vi "Raster Scan.vi"() -> ()   [LabVIEW 2012]
uses:
  Madlib.dll
panel:
  in  "XRasterRead":dbl[](array[numeric])
  in  "YRasterRead":dbl[](array[numeric])
  in  "ZRasterRead":dbl[](array[numeric])
  in  "Tab Control":T1(tab)
  in  "exportData":bool
  out "Actual Total Time":dbl format="%#.3f"
  in  "commandZ":bool
  in  "commandY":bool
  out "zRead":dbl format="%#.3g"
  out "yRead":dbl format="%#.3g"
  out "xRead":dbl format="%#.3g"
  in  "zCommand":dbl
  in  "yCommand":dbl
  in  "xCommand":dbl
  out "XY Graph":cluster{"Y":dbl[], "Y":dbl[]}[](graph)
  in  "pixel read delay":dbl=5.0
  in  "pixels reads per line":dbl=10.0
  in  "startScan":bool
  in  "3D Raster Scan":bool
  in  "mirroredMotion":bool
  in  "waveAcquistion":bool
  in  "frame delay":dbl=50.0
  in  "end of line delay":dbl=50.0
  in  "start of line delay":dbl=50.0
  in  "pixel write delay":dbl=5.0
  in  "Zend":dbl=1.0
  in  "Zstart":dbl
  in  "frames per scan":dbl=5.0
  in  "Yend":dbl=1.0
  in  "Ystart":dbl
  in  "lines per frame":dbl=10.0
  in  "pixels writes per line":dbl=20.0
  in  "Xend":dbl=1.0
  in  "Xstart":dbl
  in  "init handle":bool
  out "handle found":bool
  in  "Y-Axis Display":u8(ring)=2 items=["Point by Point", "Line", "Pixel"]
  in  "X-Axis Display":u8(ring) items=["Point by Point", "Line", "Pixel"]
  in  "stop":bool
  in  "commandX":bool
  out "Expected Total Time":dbl format="%#_6f"
  in  "exportDataSelect":u8(ring)=2 items=["ADC (blue) as graphed", "DAC (green) as graphed", "First and last ADC dpt of each line", "All pixel ADC", "All line ADC", "All frame ADC", "All pixel DAC", "All line DAC", "All frame DAC"]
  in  "Frame":u32=1 min=1
  in  "View Start of Scan ISS Commands":bool caption="View End of Scan ISS Commands"
  in  "Adv ISS Control":bool
  in  "ISSConfirm":bool
  in  "ISSReset":bool
  in  "AuxBindAxis":T2(ring)
  in  "AuxPulse":enum16{"Low to High", "High to Low"}(ring)
  in  "AuxPol":enum16{"Low", "High"}(ring)
  in  "FrameBindAxis":T2(ring)
  in  "FramePulse":enum16{"Low to High", "High to Low"}(ring)
  in  "FramePol":enum16{"Low", "High"}(ring)
  in  "LineBindAxis":T2(ring)
  in  "LinePulse":enum16{"Low to High", "High to Low"}(ring)
  in  "LinePol":enum16{"Low", "High"}(ring)
  in  "PixRestore":bool
  in  "PixBindAxis":T2(ring)
  in  "PixPulse":enum16{"Low to High", "High to Low"}(ring)
  in  "PixPol":enum16{"Low", "High"}(ring)
  in  "LineRestore":bool
  in  "FrameRestore":bool
  in  "AuxRestore":bool
  in  "PulseAux":bool
  in  "PulseFrame":bool
  in  "PulseLine":bool
  in  "PulsePix":bool
  out "zPos":dbl[](graph)
  out "yPos":dbl[](graph)
  out "xPos":dbl[](graph)
  # "Step 1: Initialize an MCL device"
  # "Step 6: Define the Scan Timing"
  # "ms"
  # "ms"
  # "ms"
  # "Step 2: Use the \"ISS Config.\" tab to set\n             up and test the ISS option."
  # "ms"
  # "ms"
  # "Step 3: Choose how to perform the scan"
  # "Step 7: Run the scan"
  # "use waveform acquisition \n(16-bit NanoDrive)"
  # "pixel axis mirrors\nmotion on return"
  # "3-D raster scan"
  # "s"
  # "Step 4: Define the region to scan"
  # "s"
  # "Nano-Drive X-Axis (pixel) scan region"
  # "Step 8: Export the data"
  # "start"
  # "um"
  # "end"
  # "um"
  # "Nano-Drive Y-Axis (line) scan region"
  # "generates a file with 2 columns of data; the left containing the graph's; X-axis, the right containing the graph'sY-axis."
  # "*"
  # "start"
  # "um"
  # "end"
  # "um"
  # "Nano-Drive Z-Axis (frame) scan region"
  # "Step 9: Release the MCL device and\n              end the VI."
  # "start"
  # "um"
  # "end"
  # "um"
  # "Step 5: Define the Scan Resolution"
  # "Graph Configuration"
  # "Current Positions"
  # "X axis"
  # "Y axis"
  # "Z axis"
  # "ISS Configuration"
  # "Pixel Clock"
  # "Line Clock"
  # "Frame Clock"
  # "Auxilary Clock"
  # "* Only one clock can be bound to an axis or event. Binding a second clock\n    replaces the first with the second"
  # "Confirm/Reset \nISS Configuration:"
  # "* Changes made here take no effect until confirmed."
  # "* Binding a Clock to an Axis will result in the suspension of live\n  position reads."
  # "Programmatic ISS Control"
  # "Pulse Individual \nISS Clocks:"
  # "* Pulsing will reset Clock to Low polarity."
  # "X\n\na\nx\ni\ns"
  # "Y\n\na\nx\ni\ns"
  # "Z\n\na\nx\ni\ns"
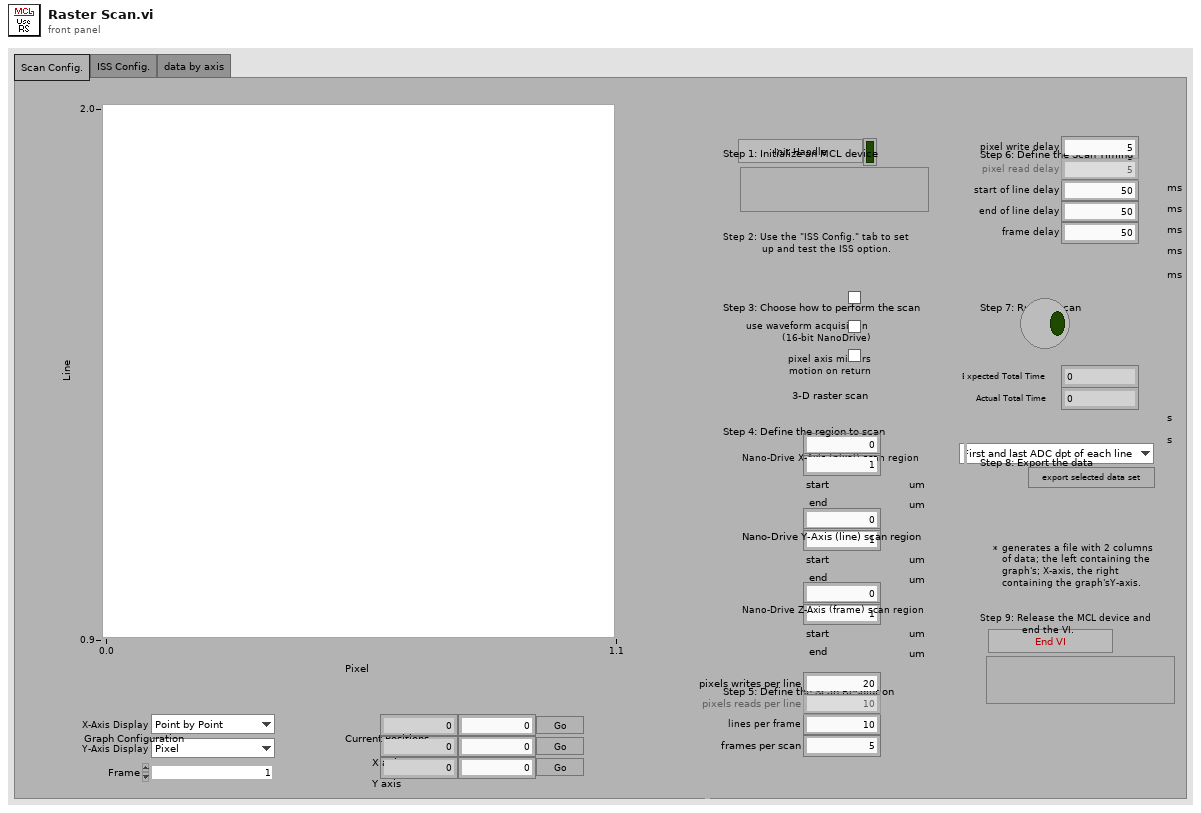
[diagram p1: front panel]
types:
  T1 = enum32{"Scan Config.", "ISS Config.", "data by axis"}
  T2 = enum16{"Unbound", "X Axis", "Y Axis", "Z Axis", "Auxilary", "Waveform Read", "Waveform Write"}
  T3 = cluster{"ISSReset":bool, "Pixel Confirmed Options":cluster{"clock (1=Pixel)":i32, "Pixel Polarity":enum16{"Low", "High"}, "Pixel Pulse":enum16{"Low to High", "High to Low"}, "Pixel Bind":enum16{"Unbound", "X Axis", "Y Axis", "Z Axis", "Auxilary", "Waveform Read", "Waveform Write"}}, "Line Confirmed Options":cluster{"clock (1=Pixel)":i32, "Pixel Polarity":enum16{"Low", "High"}, "Pixel Pulse":enum16{"Low to High", "High to Low"}, "Pixel Bind":enum16{"Unbound", "X Axis", "Y Axis", "Z Axis", "Auxilary", "Waveform Read", "Waveform Write"}}, "Frame Confirmed Options":cluster{"clock (1=Pixel)":i32, "Pixel Polarity":enum16{"Low", "High"}, "Pixel Pulse":enum16{"Low to High", "High to Low"}, "Pixel Bind":enum16{"Unbound", "X Axis", "Y Axis", "Z Axis", "Auxilary", "Waveform Read", "Waveform Write"}}, "Aux Confirmed Options":cluster{"clock (1=Pixel)":i32, "Pixel Polarity":enum16{"Low", "High"}, "Pixel Pulse":enum16{"Low to High", "High to Low"}, "Pixel Bind":enum16{"Unbound", "X Axis", "Y Axis", "Z Axis", "Auxilary", "Waveform Read", "Waveform Write"}}}
  T4 = cluster{"waveAcquistion":bool, "mirroredMotion":bool, "3D Raster Scan":bool}
  T5 = cluster{"Xstart":dbl, "Xend":dbl, "Ystart":dbl, "Yend":dbl, "Zstart":dbl, "Zend":dbl}
  T6 = cluster{"pixels writes per line":dbl, "pixels reads per line":dbl, "lines per frame":dbl, "frames per scan":dbl}
  T7 = cluster{"pixel write delay":dbl, "pixel read delay":dbl, "start of line delay":dbl, "end of line delay":dbl, "frame delay":dbl}
  T8 = cluster{"exportDataSelect":u8, "exportData":bool}
  T9 = cluster{"X-Axis Display":u8, "Y-Axis Display":u8, u32}
  T10 = cluster{cluster{"waveAcquistion":bool, "mirroredMotion":bool, "3D Raster Scan":bool}, cluster{"Xstart":dbl, "Xend":dbl, "Ystart":dbl, "Yend":dbl, "Zstart":dbl, "Zend":dbl}, cluster{"pixels writes per line":dbl, "pixels reads per line":dbl, "lines per frame":dbl, "frames per scan":dbl}, cluster{"pixel write delay":dbl, "pixel read delay":dbl, "start of line delay":dbl, "end of line delay":dbl, "frame delay":dbl}}
  T11 = cluster{"XY Graph":refnum<vi>, cluster{"exportDataSelect":u8, "exportData":bool}, cluster{"X-Axis Display":u8, "Y-Axis Display":u8, u32}}
  T12 = cluster{"PixRestore":bool, "LineRestore":bool, "FrameRestore":bool, "AuxRestore":bool}
  T13 = cluster{"PixBindAxis":enum16{"Unbound", "X Axis", "Y Axis", "Z Axis", "Auxilary", "Waveform Read", "Waveform Write"}, "LineBindAxis":enum16{"Unbound", "X Axis", "Y Axis", "Z Axis", "Auxilary", "Waveform Read", "Waveform Write"}, "FrameBindAxis":enum16{"Unbound", "X Axis", "Y Axis", "Z Axis", "Auxilary", "Waveform Read", "Waveform Write"}, "AuxBindAxis":enum16{"Unbound", "X Axis", "Y Axis", "Z Axis", "Auxilary", "Waveform Read", "Waveform Write"}}
  T14 = cluster{"PixPol":enum16{"Low", "High"}, "PixPulse":enum16{"Low to High", "High to Low"}, "LinePol":enum16{"Low", "High"}, "LinePulse":enum16{"Low to High", "High to Low"}, "FramePol":enum16{"Low", "High"}, "FramePulse":enum16{"Low to High", "High to Low"}, "AuxPol":enum16{"Low", "High"}, "AuxPulse":enum16{"Low to High", "High to Low"}}
  T15 = cluster{"PulsePix":bool, "PulseLine":bool, "PulseFrame":bool, "PulseAux":bool}
  T16 = cluster{"ISS Options":cluster{"ISSReset":bool, "Pixel Confirmed Options":cluster{"clock (1=Pixel)":i32, "Pixel Polarity":enum16{"Low", "High"}, "Pixel Pulse":enum16{"Low to High", "High to Low"}, "Pixel Bind":enum16{"Unbound", "X Axis", "Y Axis", "Z Axis", "Auxilary", "Waveform Read", "Waveform Write"}}, "Line Confirmed Options":cluster{"clock (1=Pixel)":i32, "Pixel Polarity":enum16{"Low", "High"}, "Pixel Pulse":enum16{"Low to High", "High to Low"}, "Pixel Bind":enum16{"Unbound", "X Axis", "Y Axis", "Z Axis", "Auxilary", "Waveform Read", "Waveform Write"}}, "Frame Confirmed Options":cluster{"clock (1=Pixel)":i32, "Pixel Polarity":enum16{"Low", "High"}, "Pixel Pulse":enum16{"Low to High", "High to Low"}, "Pixel Bind":enum16{"Unbound", "X Axis", "Y Axis", "Z Axis", "Auxilary", "Waveform Read", "Waveform Write"}}, "Aux Confirmed Options":cluster{"clock (1=Pixel)":i32, "Pixel Polarity":enum16{"Low", "High"}, "Pixel Pulse":enum16{"Low to High", "High to Low"}, "Pixel Bind":enum16{"Unbound", "X Axis", "Y Axis", "Z Axis", "Auxilary", "Waveform Read", "Waveform Write"}}}, cluster{"ISSConfirm":bool, "ISSReset":bool}, cluster{"PixRestore":bool, "LineRestore":bool, "FrameRestore":bool, "AuxRestore":bool}, cluster{"PixBindAxis":enum16{"Unbound", "X Axis", "Y Axis", "Z Axis", "Auxilary", "Waveform Read", "Waveform Write"}, "LineBindAxis":enum16{"Unbound", "X Axis", "Y Axis", "Z Axis", "Auxilary", "Waveform Read", "Waveform Write"}, "FrameBindAxis":enum16{"Unbound", "X Axis", "Y Axis", "Z Axis", "Auxilary", "Waveform Read", "Waveform Write"}, "AuxBindAxis":enum16{"Unbound", "X Axis", "Y Axis", "Z Axis", "Auxilary", "Waveform Read", "Waveform Write"}}, cluster{"PixPol":enum16{"Low", "High"}, "PixPulse":enum16{"Low to High", "High to Low"}, "LinePol":enum16{"Low", "High"}, "LinePulse":enum16{"Low to High", "High to Low"}, "FramePol":enum16{"Low", "High"}, "FramePulse":enum16{"Low to High", "High to Low"}, "AuxPol":enum16{"Low", "High"}, "AuxPulse":enum16{"Low to High", "High to Low"}}, cluster{"PulsePix":bool, "PulseLine":bool, "PulseFrame":bool, "PulseAux":bool}, "handle":i32}
  T17 = cluster{"XRasterRead":dbl[], "YRasterRead":dbl[], "ZRasterRead":dbl[]}
  T18 = cluster{"stop":refnum<vi>, "startScan":refnum<vi>, "Adv ISS Control":bool}
  T19 = cluster{refnum<vi>, "handle":i32, "OwningVI":refnum<vi>}
  T20 = cluster{"reset pixel":bool, "reset line":bool, "reset frame":bool, "reset aux":bool}
  T21 = cluster{cluster{"stop":refnum<vi>, "startScan":refnum<vi>, "Adv ISS Control":bool}, cluster{refnum<vi>, "handle":i32, "OwningVI":refnum<vi>}}
  T22 = cluster{"X Command Ramp":dbl[], "Y Command Ramp":dbl[], "Z Command Ramp":dbl[]}
  T23 = cluster{"Options":cluster{"waveAcquistion":bool, "mirroredMotion":bool, "3DRasterScan":bool}, "Regions":cluster{"xStart":dbl, "xEnd":dbl, "yStart":dbl, "yEnd":dbl, "zStart":dbl, "zEnd":dbl}, "Resolution":cluster{"pixelsWritesPerLine":dbl, "pixelsReadsPerLine":dbl, "linesPerFrame":dbl, "framesPerScan":dbl}, "Timing":cluster{"pixelWriteDelay":dbl, "pixelReadDelay":dbl, "startOfLineDelay":dbl, "endOfLineDelay":dbl, "frameDelay":dbl}}
  T24 = cluster{refnum<vi>[], refnum<vi>[], refnum<vi>[]}
  T25 = cluster{"clock (1=Pixel)":i32, "Pixel Polarity":enum16{"Low", "High"}, "Pixel Pulse":enum16{"Low to High", "High to Low"}, "Pixel Bind":enum16{"Unbound", "X Axis", "Y Axis", "Z Axis", "Auxilary", "Waveform Read", "Waveform Write"}}
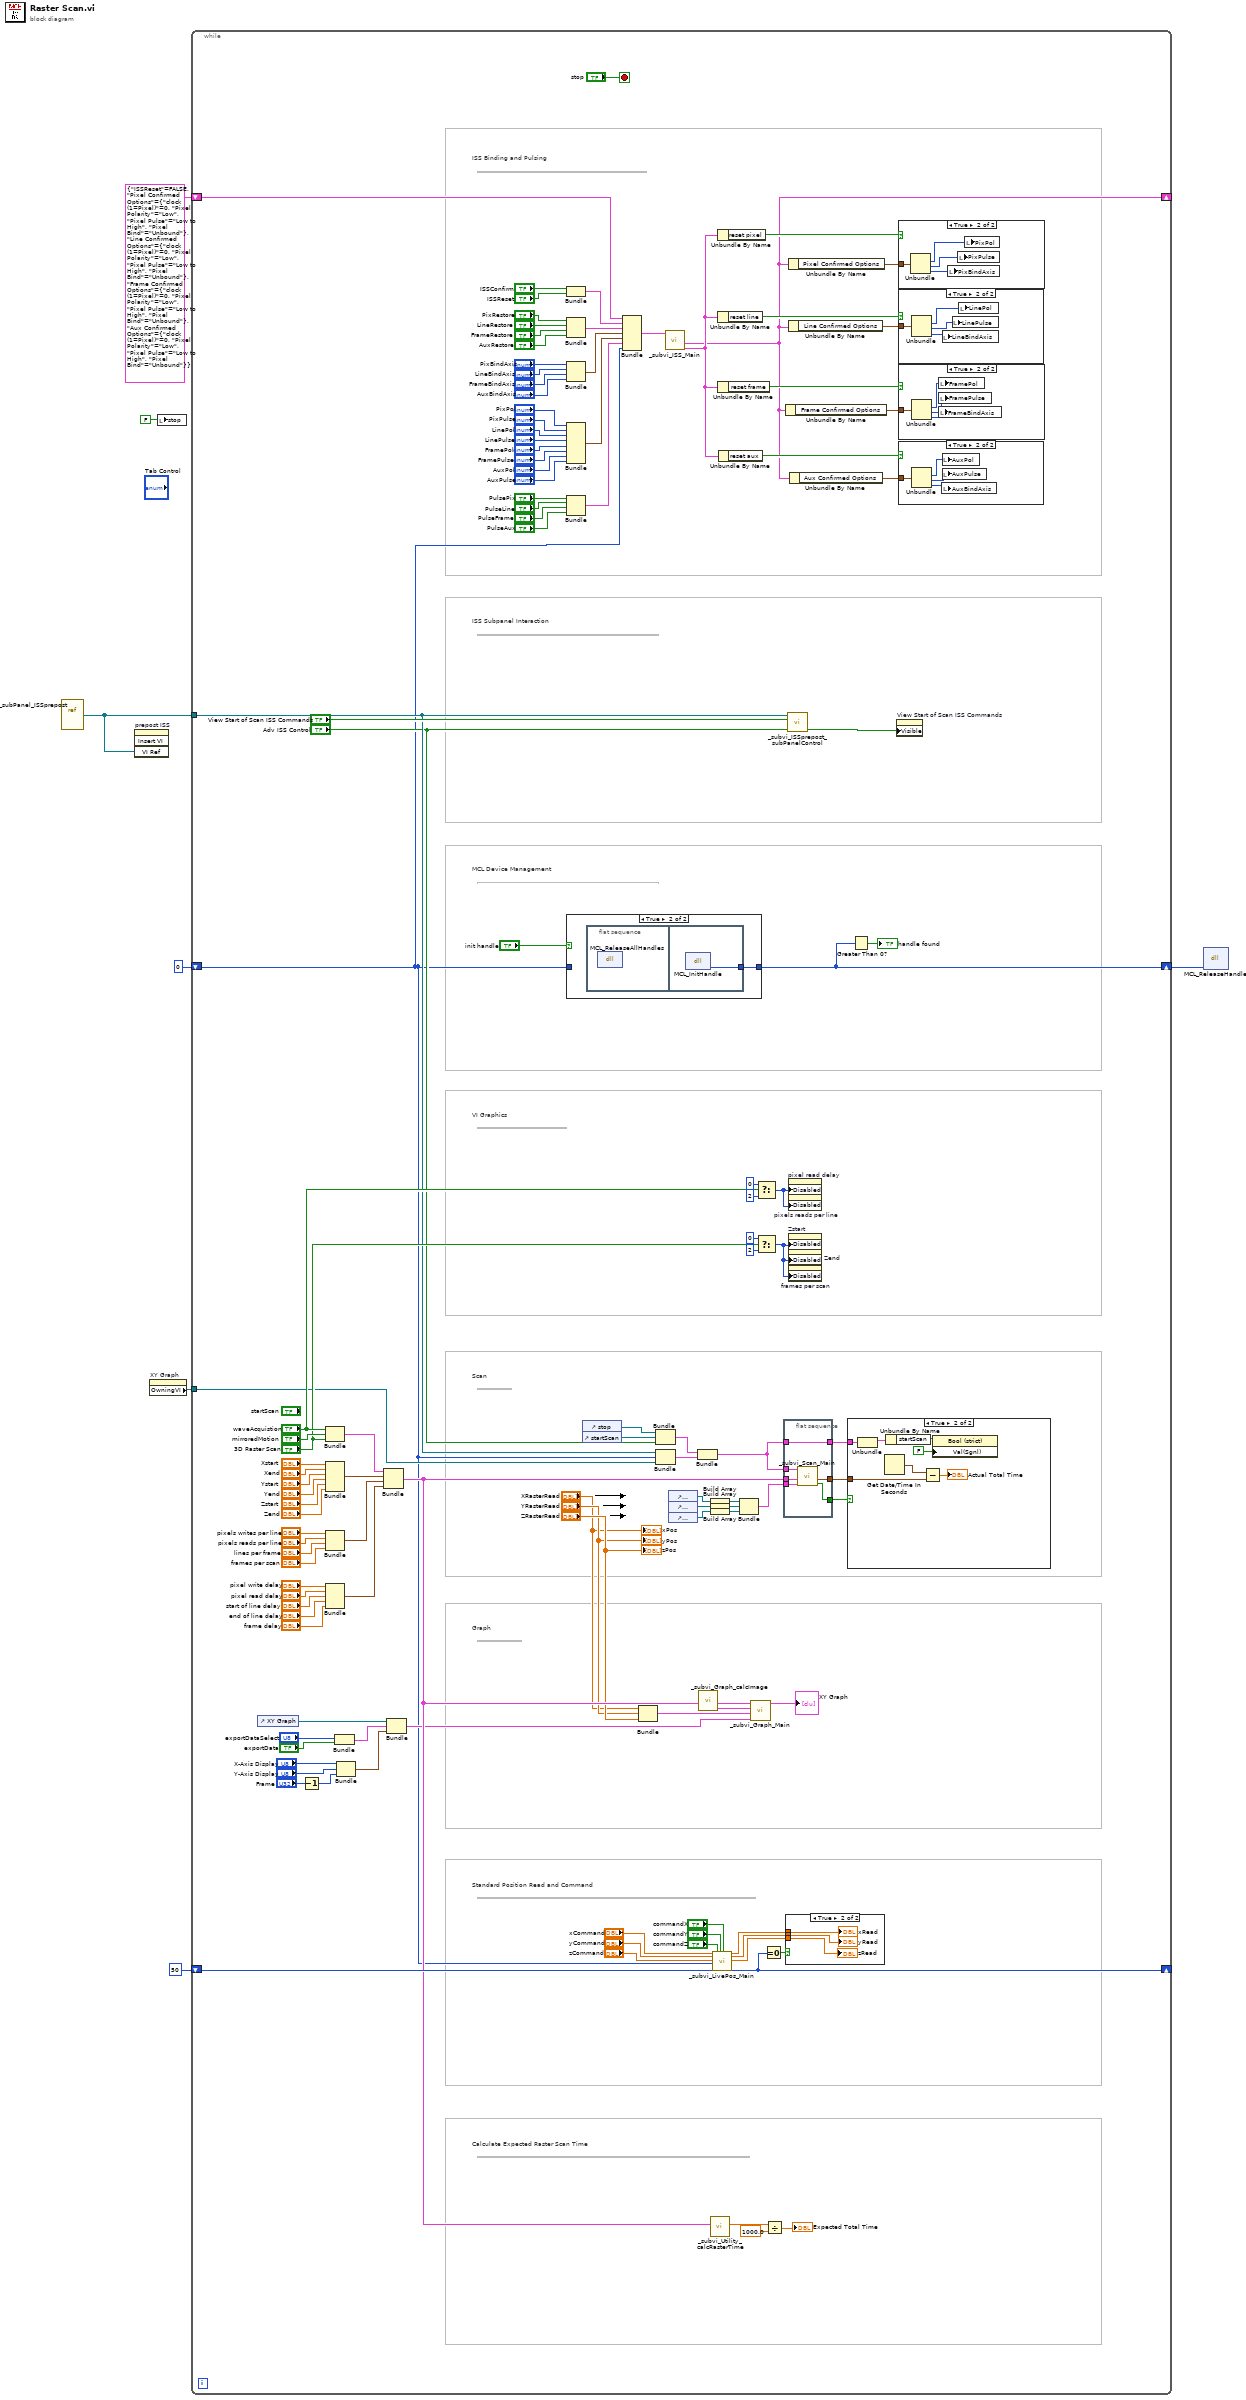
[diagram p0: block diagram]
diagram:
  n1 = vi-ref "_subPanel_ISSprepost.vi"() -> (w5:refnum<vi>)
  n2 = invoke on="prepost ISS" class="SubPanel" method="Insert VI"("VI Ref"=w5) -> ()  [unwired: 3 in, 4 out]
  n3 = property on="XY Graph" class="XYGraph (strict)"() -> ("OwningVI"=w2:refnum<vi>)  [unwired: 2 in, 2 out]
  n4 = local write "stop"(FALSE ("stop")) -> ()
  n5 = while {
    shift-right: [w95] -> _
    shift-left: T3 {"ISSReset"=FALSE, "Pixel Confirmed Options"={"clock (1=Pixel)"=0, "Pixel Polarity"=enum."Low", "Pixel Pulse"=enum."Low to High", "Pixel Bind"=enum."Unbound"}, "Line Confirmed Options"={"clock (1=Pixel)"=0, "Pixel Polarity"=enum."Low", "Pixel Pulse"=enum."Low to High", "Pixel Bind"=enum."Unbound"}, "Frame Confirmed Options"={"clock (1=Pixel)"=0, "Pixel Polarity"=enum."Low", "Pixel Pulse"=enum."Low to High", "Pixel Bind"=enum."Unbound"}, "Aux Confirmed Options"={"clock (1=Pixel)"=0, "Pixel Polarity"=enum."Low", "Pixel Pulse"=enum."Low to High", "Pixel Bind"=enum."Unbound"}} ("ISS Options") -> [w61]
    tunnel: w5 -> [w56]
    shift-right: [w89] -> w4
    shift-left: 0 ("handle") -> [w8]
    tunnel: w2 -> [w54]
    shift-right: [w31] -> _
    shift-left: u32 50 ("axis") -> [w33]
    stop <- "stop" stop-if-true
    # "Calculate Expected Raster Scan Time"
    # "Standard Position Read and Command"
    # "Graph"
    # "Scan"
    # "VI Graphics"
    # "MCL Device Management"
    # "ISS Subpanel Interaction"
    # "ISS Binding and Pulsing"
    n6 = control-ref of="XY Graph"() -> (w60:refnum<vi>)
    n7 = Decrement(x="Frame") -> (x-1=w10:u32)
    n8 = Bundle("waveAcquistion"="waveAcquistion", "mirroredMotion"="mirroredMotion", "3D Raster Scan"="3D Raster Scan") -> (w65:T4)  [unwired: 1 out]
    n9 = Bundle("Xstart"="Xstart", "Xend"="Xend", "Ystart"="Ystart", "Yend"="Yend", "Zstart"="Zstart", "Zend"="Zend") -> (w64:T5)  [unwired: 1 out]
    n10 = Bundle("pixels writes per line"="pixels writes per line", "pixels reads per line"="pixels reads per line", "lines per frame"="lines per frame", "frames per scan"="frames per scan") -> (w63:T6)  [unwired: 1 out]
    n11 = Bundle("pixel write delay"="pixel write delay", "pixel read delay"="pixel read delay", "start of line delay"="start of line delay", "end of line delay"="end of line delay", "frame delay"="frame delay") -> (w62:T7)  [unwired: 1 out]
    n12 = Bundle("exportDataSelect"="exportDataSelect", "exportData"="exportData") -> (w24:T8)  [unwired: 1 out]
    n13 = Bundle("X-Axis Display"="X-Axis Display", "Y-Axis Display"="Y-Axis Display", w10) -> (w27:T9)  [unwired: 1 out]
    n14 = Bundle(w65, w64, w63, w62) -> (w19:T10)  [unwired: 1 out]
    n15 = Bundle("XY Graph"=w60, w24, w27) -> (w16:T11)  [unwired: 1 out]
    n16 = Bundle("ISSConfirm"="ISSConfirm", "ISSReset"="ISSReset") -> (w101:cluster{"ISSConfirm":bool, "ISSReset":bool})  [unwired: 1 out]
    n17 = Bundle("PixRestore"="PixRestore", "LineRestore"="LineRestore", "FrameRestore"="FrameRestore", "AuxRestore"="AuxRestore") -> (w100:T12)  [unwired: 1 out]
    n18 = Bundle("PixBindAxis"="PixBindAxis", "LineBindAxis"="LineBindAxis", "FrameBindAxis"="FrameBindAxis", "AuxBindAxis"="AuxBindAxis") -> (w99:T13)  [unwired: 1 out]
    n19 = Bundle("PixPol"="PixPol", "PixPulse"="PixPulse", "LinePol"="LinePol", "LinePulse"="LinePulse", "FramePol"="FramePol", "FramePulse"="FramePulse", "AuxPol"="AuxPol", "AuxPulse"="AuxPulse") -> (w98:T14)  [unwired: 1 out]
    n20 = Bundle("PulsePix"="PulsePix", "PulseLine"="PulseLine", "PulseFrame"="PulseFrame", "PulseAux"="PulseAux") -> (w97:T15)  [unwired: 1 out]
    n21 = case shown="True" "init handle" {
      tunnel: [w149 w150] -> w89
      tunnel: w8 -> [w149 _]
      frame False {
      }
      frame True {
        n22 = flat-sequence {
          tunnel: [w151] -> w150
          frame #0 {
            n23 = dll-call lib="C:/Users/Labview/Desktop/SRR/Madlib_x64/Labview Examples/MADLib.dll" fn="MCL_ReleaseAllHandles" label="Release All Handles"() -> ()  [unwired: 3 in, 3 out]
          }
          frame #1 {
            n24 = dll-call lib="C:/Users/Labview/Desktop/SRR/Madlib_x64/Labview Examples/Madlib.dll" fn="MCL_InitHandle" label="Init Handle"() -> ("handle"=w151:i32)  [unwired: 3 in, 2 out]
          }
        }
      }
    }
    n25 = control-ref of="stop"() -> (w49:refnum<vi>)
    n26 = control-ref of="startScan"() -> (w50:refnum<vi>)
    n27 = Bundle("ISS Options"=w61, w101, w100, w99, w98, w97, "handle"=w8) -> (w96:T16)  [unwired: 1 out]
    n28 = Bundle("XRasterRead"="XRasterRead", "YRasterRead"="YRasterRead", "ZRasterRead"="ZRasterRead") -> (w15:T17)  [unwired: 1 out]
    n29 = Bundle("stop"=w49, "startScan"=w50, "Adv ISS Control"="Adv ISS Control") -> (w52:T18)  [unwired: 1 out]
    n30 = Bundle(w56, "handle"=w8, "OwningVI"=w54) -> (w51:T19)  [unwired: 1 out]
    n31 = call "_subvi_ISS_Main.vi"("ISS Options"=w96) -> ("ISS Reset"=w128:T20, "ISS Options OUT"=w95:T3)  [unwired: 9 out]
    n32 = control-ref of="XRasterRead"() -> (w22:refnum<vi>)
    n33 = control-ref of="YRasterRead"() -> (w21:refnum<vi>)
    n34 = control-ref of="ZRasterRead"() -> (w20:refnum<vi>)
    n35 = Bundle(w52, w51) -> (w28:T21)  [unwired: 1 out]
    n36 = call "_subvi_Graph_calcImage.vi"("Scan Parameters IN"=w19) -> ("AllDAC"=w17:T22, "Scan Parameters"=w18:T23)  [unwired: 1 in, 8 out]
    n37 = Build Array(w22) -> (w46:refnum<vi>[])
    n38 = Build Array(w21) -> (w47:refnum<vi>[])
    n39 = Build Array(w20) -> (w48:refnum<vi>[])
    n40 = call "_subvi_Utility_calcRasterTime.vi"("NewScan"=w19) -> ("totalRasterTime"=w36:dbl)  [unwired: 10 out]
    n41 = call "_subvi_LivePos_Main.vi"("xCommand"="xCommand", "yCommand"="yCommand", "zCommand"="zCommand", "handle"=w8, "counter"=w33, "commandZ"="commandZ", "commandY"="commandY", "commandX"="commandX") -> ("xRead"=w45:dbl, "yRead"=w44:dbl, "zRead"=w43:dbl, "counter"=w31:u32)  [unwired: 8 out]
    n42 = Unbundle By Name(w128) -> ("reset pixel"=w132:bool)
    n43 = Unbundle By Name(w128) -> ("reset line"=w131:bool)
    n44 = Unbundle By Name(w128) -> ("reset frame"=w130:bool)
    n45 = Unbundle By Name(w128) -> ("reset aux"=w129:bool)
    n46 = Bundle(w46, w47, w48) -> (w53:T24)  [unwired: 1 out]
    n47 = call "_subvi_Graph_Main.vi"("GraphOptions"=w16, "AllADC"=w15, "AllDAC"=w17, "ScanParameters"=w18) -> ("Image Graph"=→"XY Graph":cluster{dbl[], dbl[]}[])  [unwired: 7 out]
    n48 = Select(t=u8 0 ("Disabled"), s="waveAcquistion", f=u8 2) -> (s? t:f=w84:u8)
    n49 = Select(t=u8 0 ("Disabled"), s="3D Raster Scan", f=u8 2) -> (s? t:f=w57:u8)
    n50 = Equal To 0?(x=w31) -> (x = 0?=w32:bool)
    n51 = Divide(x=w36, y=1000.0) -> (x/y=→"Expected Total Time":dbl)
    n52 = flat-sequence {
      tunnel: w53 -> [w138]
      tunnel: w19 -> [w137]
      tunnel: [w136] -> w30
      tunnel: w28 -> [w135]
      tunnel: [w134] -> w29
      tunnel: w28 -> [w134]
      tunnel: [w133] -> w23
      frame #0 {
        n53 = call "_subvi_Scan_Main.vi"("IndicatorReferenceArrays"=w138, "NewScan"=w137, "MainViReferences"=w135) -> ("finished"=w136:bool, "startTimeOfScan"=w133:timestamp)  [unwired: 7 out]
      }
    }
    n54 = Unbundle By Name(w95) -> ("Frame Confirmed Options"=w125:T25)
    n55 = case shown="True" w32 {
      tunnel: w45 -> [_ w148]
      tunnel: w44 -> [_ w147]
      tunnel: w43 -> [_ w146]
      frame False {
      }
      frame True {
        "xRead" <- w148
        "yRead" <- w147
        "zRead" <- w146
      }
    }
    n56 = call "_subvi_ISSprepost_subPanelControl.vi"("Adv ISS Control"="Adv ISS Control", "View Start of Scan ISS Commands"="View Start of Scan ISS Commands", "VI Refnum"=w56) -> ("Show Advanced Options"=w92:bool)  [unwired: 8 out]
    n57 = Unbundle By Name(w95) -> ("Pixel Confirmed Options"=w127:T25)
    n58 = Unbundle By Name(w95) -> ("Line Confirmed Options"=w126:T25)
    n59 = property on="pixel read delay" class="DigNum (strict)"("Disabled"=w84) -> ()  [unwired: 2 in, 2 out]
    n60 = property on="pixels reads per line" class="DigNum (strict)"("Disabled"=w84) -> ()  [unwired: 2 in, 2 out]
    n61 = property on="Zstart" class="DigNum (strict)"("Disabled"=w57) -> ()  [unwired: 2 in, 2 out]
    n62 = property on="Zend" class="DigNum (strict)"("Disabled"=w57) -> ()  [unwired: 2 in, 2 out]
    n63 = property on="frames per scan" class="DigNum (strict)"("Disabled"=w57) -> ()  [unwired: 2 in, 2 out]
    n64 = Unbundle By Name(w95) -> ("Aux Confirmed Options"=w124:T25)
    n65 = case shown="True" w30 {
      tunnel: w29 -> [_ w140]
      tunnel: w23 -> [_ w139]
      frame False {
      }
      frame True {
        n66 = Unbundle(w140) -> (w142:T18)  [unwired: 1 out]
        n67 = Get Date/Time In Seconds() -> (seconds since 1Jan1904=w144:timestamp)
        n68 = Unbundle By Name(w142) -> ("startScan"=w143:refnum<vi>)
        n69 = Subtract(x=w144, y=w139) -> (x-y=→"Actual Total Time":dbl)
        n70 = property class="Bool (strict)"(reference=w143, "Val(Sgnl)"=FALSE ("Value (Signaling)")) -> ()  [unwired: 1 in, 2 out]
      }
    }
    n71 = Greater Than 0?(x=w89) -> (x > 0?=→"handle found":bool)
    n72 = property on="View Start of Scan ISS Commands" class="Bool (strict)"("Visible"=w92) -> ()  [unwired: 2 in, 2 out]
    n73 = case shown="True" w132 {
      tunnel: w127 -> [_ w164]
      frame False {
      }
      frame True {
        n74 = Unbundle(w164) -> ("Pixel Polarity"=w167:enum16{"Low", "High"}, "Pixel Pulse"=w166:enum16{"Low to High", "High to Low"}, "Pixel Bind"=w165:T2)  [unwired: 1 out]
        n75 = local write "PixBindAxis"(w165) -> ()
        n76 = local write "PixPulse"(w166) -> ()
        n77 = local write "PixPol"(w167) -> ()
      }
    }
    n78 = case shown="True" w131 {
      tunnel: w126 -> [_ w160]
      frame False {
      }
      frame True {
        n79 = Unbundle(w160) -> ("Pixel Polarity"=w161:enum16{"Low", "High"}, "Pixel Pulse"=w162:enum16{"Low to High", "High to Low"}, "Pixel Bind"=w163:T2)  [unwired: 1 out]
        n80 = local write "LineBindAxis"(w163) -> ()
        n81 = local write "LinePulse"(w162) -> ()
        n82 = local write "LinePol"(w161) -> ()
      }
    }
    n83 = case shown="True" w130 {
      tunnel: w125 -> [_ w156]
      frame False {
      }
      frame True {
        n84 = Unbundle(w156) -> ("Pixel Polarity"=w159:enum16{"Low", "High"}, "Pixel Pulse"=w158:enum16{"Low to High", "High to Low"}, "Pixel Bind"=w157:T2)  [unwired: 1 out]
        n85 = local write "FrameBindAxis"(w157) -> ()
        n86 = local write "FramePol"(w159) -> ()
        n87 = local write "FramePulse"(w158) -> ()
      }
    }
    n88 = case shown="True" w129 {
      tunnel: w124 -> [_ w152]
      frame False {
      }
      frame True {
        n89 = Unbundle(w152) -> ("Pixel Polarity"=w155:enum16{"Low", "High"}, "Pixel Pulse"=w154:enum16{"Low to High", "High to Low"}, "Pixel Bind"=w153:T2)  [unwired: 1 out]
        n90 = local write "AuxBindAxis"(w153) -> ()
        n91 = local write "AuxPol"(w155) -> ()
        n92 = local write "AuxPulse"(w154) -> ()
      }
    }
    "zPos" <- "ZRasterRead"
    "xPos" <- "XRasterRead"
    "yPos" <- "YRasterRead"
  }
  n93 = dll-call lib="C:/Users/Labview/Desktop/SRR/Madlib_x64/Labview Examples/MADLib.dll" fn="MCL_ReleaseHandle" label="Release Handle"("handle"=w4) -> ()  [unwired: 4 in, 3 out]
